vi "robotimageprocessing2.vi"(0 "Image In":T1, 7 "error in":errorcluster) -> (20 "Image Out":T1, 21 "Number of Matches (Shape Matching 1)":i32, 22 "Shape Report (Shape Matching 1)":T2(array[cluster]) {"Score" format="%.2f"; "Centroid"."y" format="%.2f"; "Centroid"."x" format="%.2f"}, 23 "Shape Report (calibrated) (Shape Matching 1)":T2(array[cluster]) {"Score" format="%.2f"; "Centroid"."y" format="%.2f"; "Centroid"."x" format="%.2f"}, 27 "error out":errorcluster)   [LabVIEW 2015]
uses:
  <vilib>/vision/Image Controls.llb/IMAQ Image.ctl
  <vilib>/vision/NI_Vision_Development_Module.lvlib
panel:
  out "file or folder exists?":bool
  out "Image Out 2":T1(plugin-control)
  out "error out 2":errorcluster
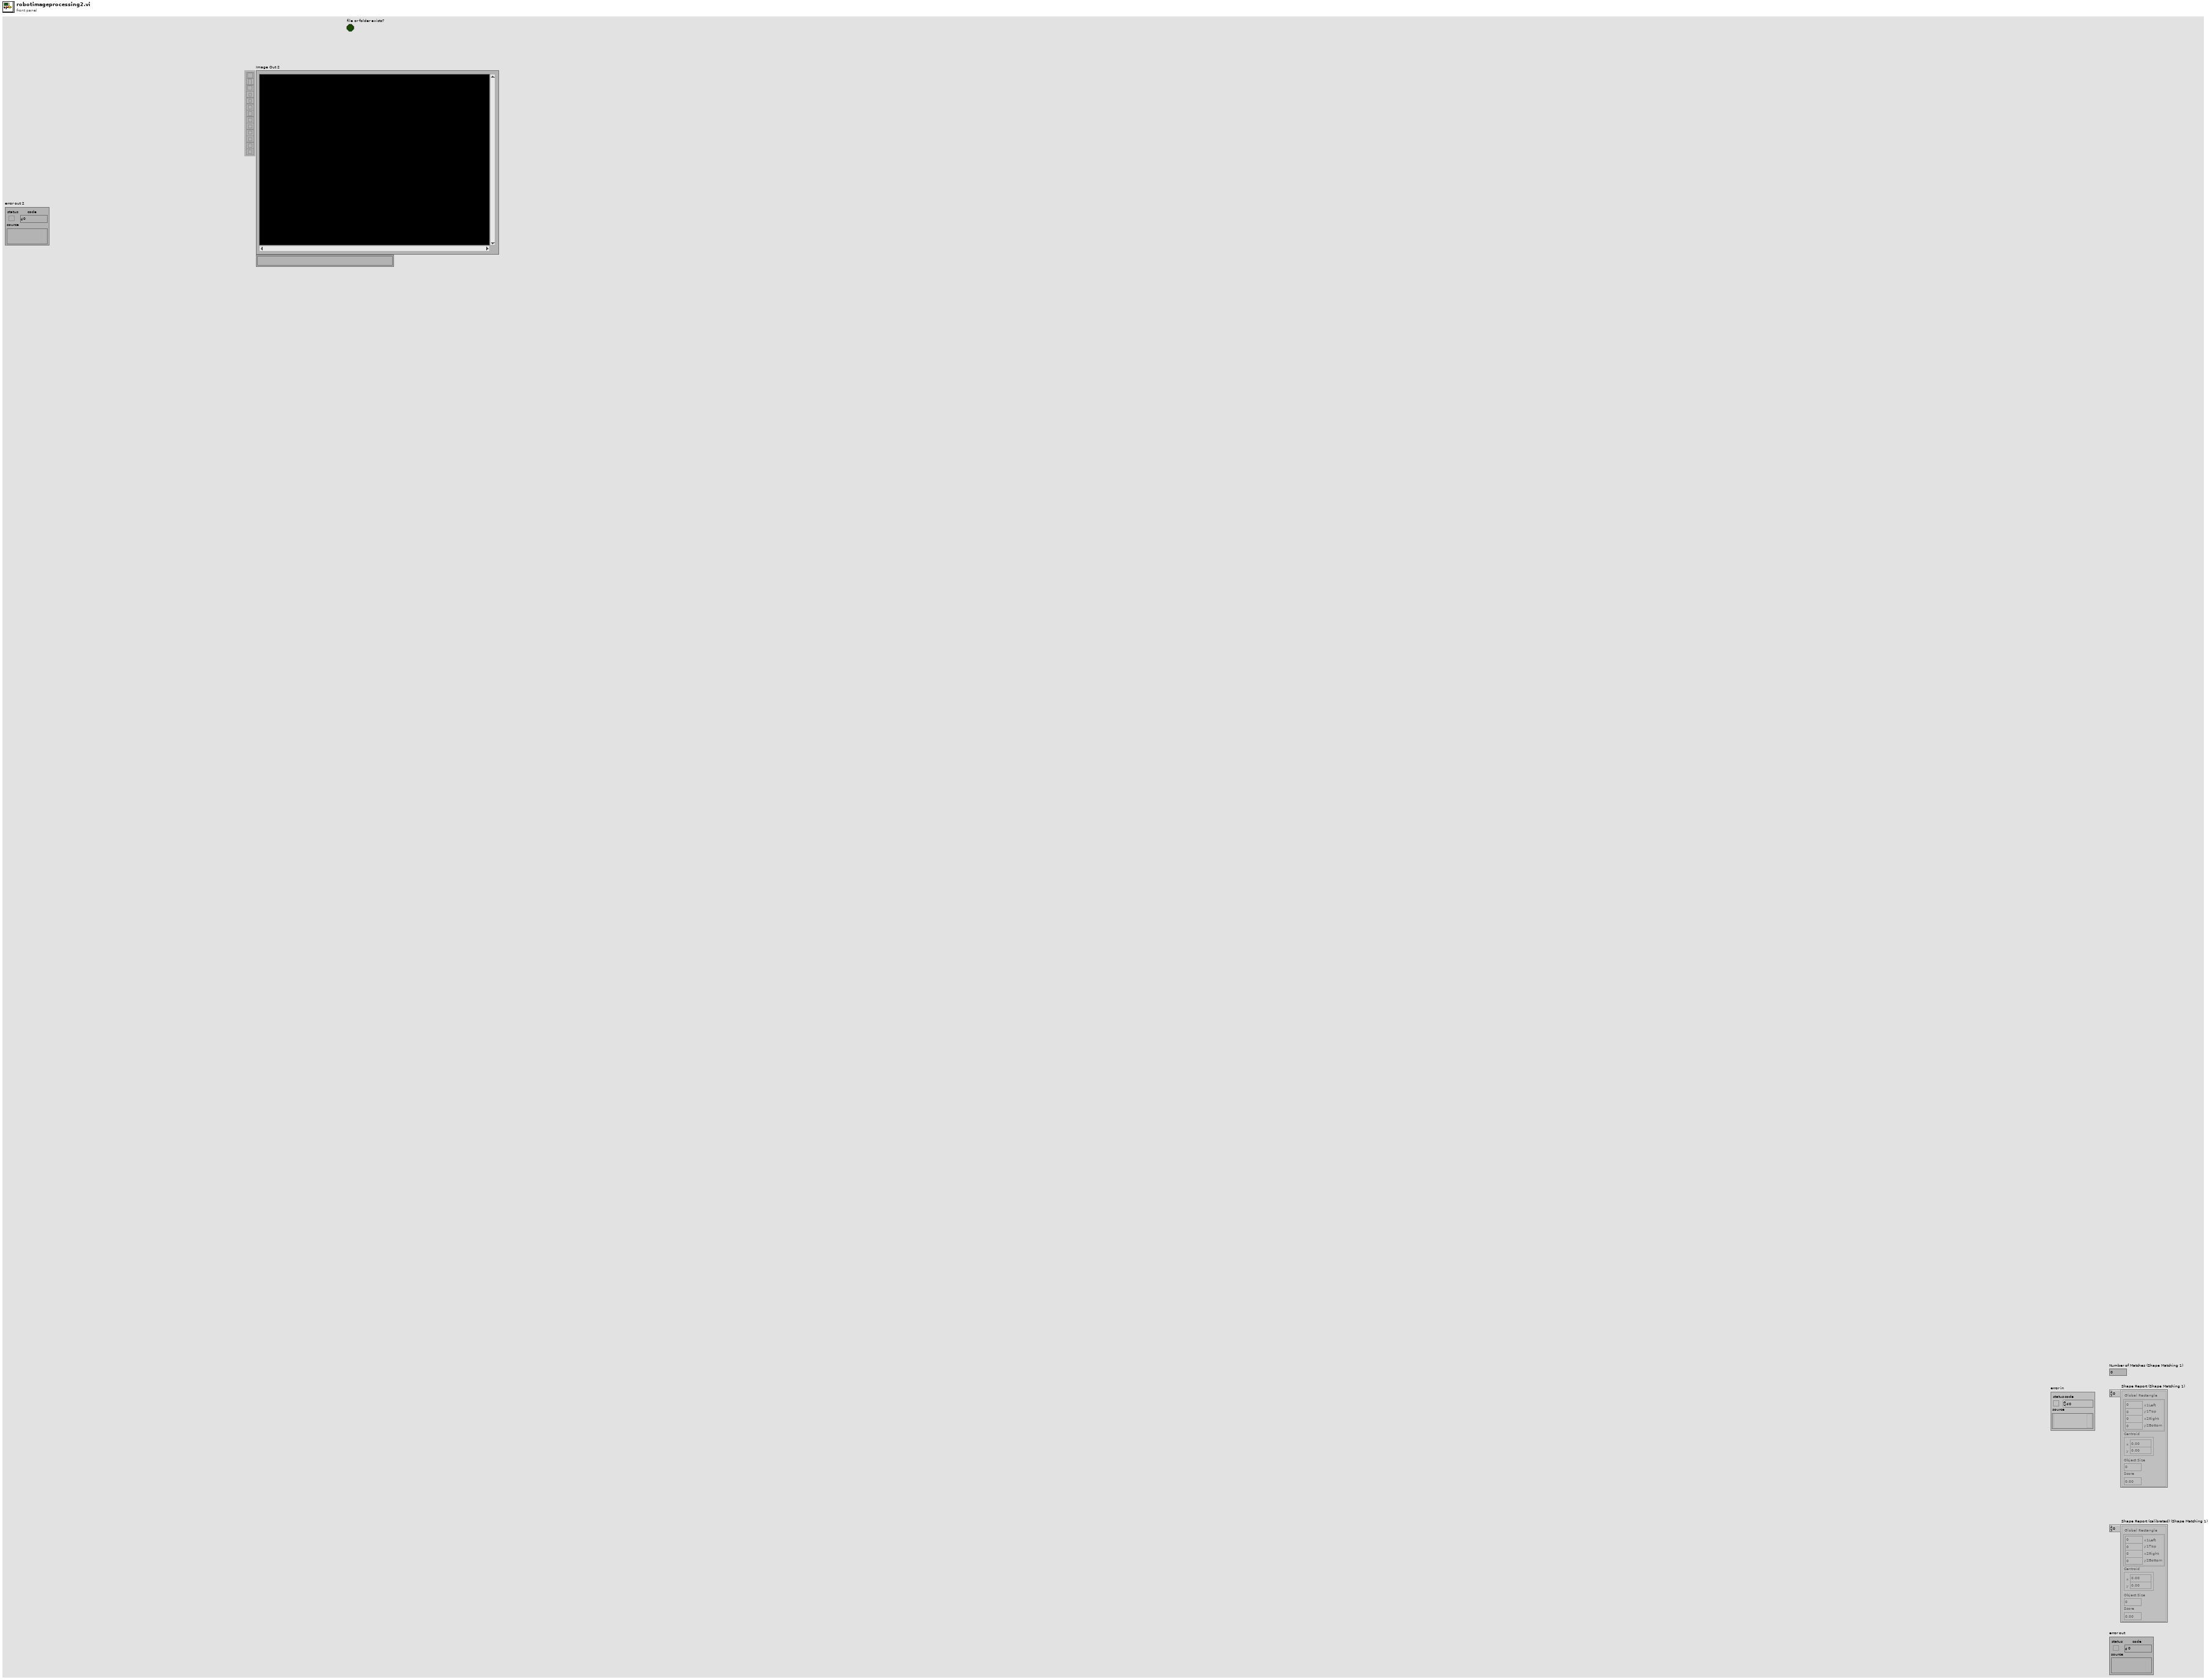
[diagram p1: front panel]
types:
  T1 = typedef "IMAQ Image.ctl" = refnum<image>
  T2 = cluster{"Global Rectangle":cluster{"x1Left":i32, "y1Top":i32, "x2Right":i32, "y2Bottom":i32}, "Centroid":cluster{"x":sgl, "y":sgl}, "Object Size":u32, "Score":dbl}[]
  T3 = enum32{"AutoM", "Close", "Dilate", "Erode", "Gradient", "Gradient out", "Gradient in", "Hit miss", "Open", "PClose", "POpen", "Thick", "Thin"}
  T4 = cluster{"Measurement Parameter":i32, "Range Lower Value":dbl, "Range Upper Value":dbl, "Range":bool, "Measurement Type":bool}[]
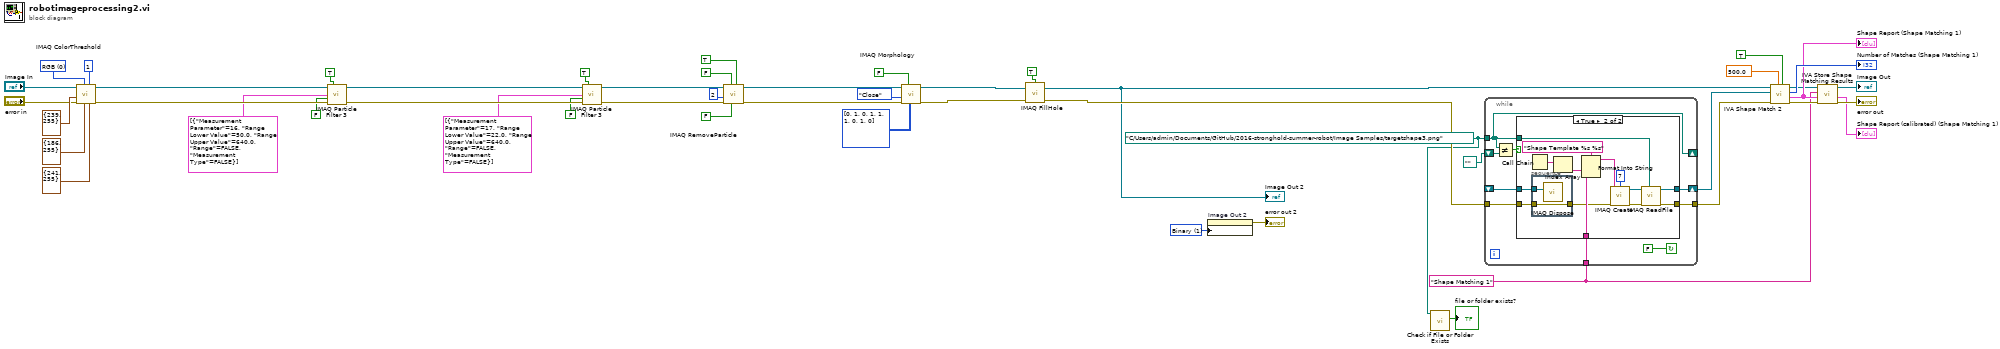
[diagram p0: block diagram]
diagram:
  w5 = u32 1 items=["Grayscale", "Binary", "Gradient", "Rainbow", "Temperature", "User Defined", "Binary 16 Bit", "Gradient 16 Bit", "Rainbow 16 Bit", "Temperature 16 Bit", "User Defined 16 Bit"] ("Palette Type")
  w7 = "Shape Matching 1" ("Step Name")
  w3 = path "C:/Users/admin/Documents/GitHub/2016-stronghold-summer-robot/Image Samples/targetshape3.png" ("Template Path")
  w49 = u16 0 items=["RGB", "HSL", "HSV", "HSI"] ("Color Mode")
  n1 = call "IMAQ ColorThreshold"("Blue or Luma or Val or Inten Range"=cluster{"Lower value":i32, "Upper value":i32} {"Lower value"=241, "Upper value"=255}, "Replace Value"=1, "Green or Sat Range"=cluster{"Lower value":i32, "Upper value":i32} {"Lower value"=186, "Upper value"=255}, "Color Mode"=w49, "error in (no error)"="error in", "Red or Hue Range"=cluster{"Lower value":i32, "Upper value":i32} {"Lower value"=239, "Upper value"=255}, "Image Src"="Image In") -> ("error out"=w43:errorcluster, "Image Dst Out"=w39:T1)  [unwired: 1 in, 2 out]
  n2 = call "IMAQ Particle Filter 3"("Image Src"=w39, "Connectivity 4/8 (8)"=TRUE, "Selection Values"=T4 [{"Measurement Parameter"=16, "Range Lower Value"=50.0, "Range Upper Value"=640.0, "Range"=FALSE, "Measurement Type"=FALSE}], "Keep/Remove Particles (F)"=FALSE ("Keep/Remove Particles"), "error in (no error)"=w43) -> ("Image Dst Out"=w34:T1, "error out"=w40:errorcluster)  [unwired: 4 in, 5 out]
  n3 = call "IMAQ Particle Filter 3"("Image Src"=w34, "Connectivity 4/8 (8)"=TRUE, "Selection Values"=T4 [{"Measurement Parameter"=17, "Range Lower Value"=22.0, "Range Upper Value"=640.0, "Range"=FALSE, "Measurement Type"=FALSE}], "Keep/Remove Particles (F)"=FALSE ("Keep/Remove Particles"), "error in (no error)"=w40) -> ("Image Dst Out"=w28:T1, "error out"=w35:errorcluster)  [unwired: 4 in, 5 out]
  n4 = call "IMAQ RemoveParticle"("Connectivity 4/8 (8)"=TRUE, "Low Pass/High Pass (Low)"=FALSE, "Square/Hexa (Square)"=FALSE, "error in (no error)"=w35, "Number of Erosion"=2, "Image Src"=w28) -> ("error out"=w27:errorcluster, "Image Dst Out"=w23:T1)  [unwired: 1 in, 3 out]
  n5 = call "IMAQ Morphology"("Structuring Element"=i32[][] [[0, 1, 0], [1, 1, 1], [0, 1, 0]], "Square/Hexa (Square)"=FALSE, "error in (no error)"=w27, "Operation"=T3."Close", "Image Src"=w23) -> ("error out"=w22:errorcluster, "Image Dst Out"=w20:T1)  [unwired: 2 in, 3 out]
  n6 = call "IMAQ FillHole"("error in (no error)"=w22, "Image Src"=w20, "Connectivity 4/8 (8)"=TRUE) -> ("error out"=w19:errorcluster, "Image Dst Out"=w4:T1)  [unwired: 1 in, 2 out]
  "Image Out 2" <- w4
  n7 = property on="Image Out 2" class="ImageControl"("Palette:Palette Type"=w5) -> (error out=→"error out 2":errorcluster)  [unwired: 2 in, 1 out]
  n8 = call <vilib>:"Check if File or Folder Exists.vi"("path"=w3) -> ("file or folder exists?"=→"file or folder exists?":bool)  [unwired: 8 in, 2 out]
  n9 = while {
    shift-right: [w59] -> w8
    shift-left: _ -> [w58]
    tunnel: [w56] -> w9
    tunnel: w19 -> [w55]
    tunnel: w3 -> [w53]
    tunnel: w7 -> [w54]
    shift-right: [w53] -> _
    shift-left: path "" ("Template Path") -> [w52]
    stop <- FALSE continue-if-true
    n10 = Not Equal?(x=w53, y=w52) -> (x != y?=w51:bool)
    n11 = case shown="True" w51 {
      tunnel: [w61 w72] -> w59
      tunnel: w58 -> [w61 w65]
      tunnel: [w60 w70] -> w56
      tunnel: w55 -> [w60 w64]
      tunnel: w53 -> [_ w62]
      tunnel: w54 -> [_ w66]
      frame False {
      }
      frame True {
        n12 = Call Chain() -> (call chain=w68:string[])
        n13 = stacked-sequence {
          tunnel: w65 -> [w77]
          tunnel: w64 -> [w76]
          tunnel: [w76] -> w63
          frame #0 {
            n14 = call "IMAQ Dispose"("Image"=w77) -> ()  [unwired: 2 in, 4 out]
          }
        }
        n15 = Index Array(array=w68) -> (element=w67:string)  [unwired: 1 in]
        n16 = Format Into String(format string="Shape Template %s %s" ("Image Name"), w67, w66) -> (resulting string=w75:string)  [unwired: 2 in, 1 out]
        n17 = call "IMAQ Create"("Border Size"=7, "Image Name"=w75, "error in (no error)"=w63) -> ("New Image"=w73:T1, "error out"=w71:errorcluster)  [unwired: 1 in, 1 out]
        n18 = call "IMAQ ReadFile"("File Path"=w62, "error in (no error)"=w71, "Image"=w73) -> ("error out"=w70:errorcluster, "Image Out"=w72:T1)  [unwired: 2 in, 5 out]
      }
    }
  }
  n19 = call <vilib>:"IVA Shape Match 2.vi"("Scale Invariance"=TRUE, "Minimal Score"=500.0, "error in (no error)"=w9, "Template"=w8, "Image Src"=w4) -> ("error out"=w15:errorcluster, "Shape Report"=w13:T2, "Number of Matches"=→"Number of Matches (Shape Matching 1)":i32, "Image Out"=w12:T1)  [unwired: 3 out]
  "Shape Report (Shape Matching 1)" <- w13
  n20 = call <vilib>:"IVA Store Shape Matching Results.vi"("error in (no error)"=w15, "Shape Report"=w13, "Step Name"=w7, "Image in"=w12) -> ("error out"=→"error out":errorcluster, "Shape Report (calibrated)"=→"Shape Report (calibrated) (Shape Matching 1)":T2, "Image dup"=→"Image Out":T1)  [unwired: 5 out]
